vi "Check Can Uninit.vi"(8 "Error in":errorcluster, 10 "Actor in":refnum<class "Actor.lvclass">) -> (1 "Uninit":bool, 2 "Actor out":refnum<class "Actor.lvclass">)   [LabVIEW 2020, in "jettl.lvlib" / "Actor.lvlib"]
uses:
  Actor.lvlib
  Actor/Actor.lvclass
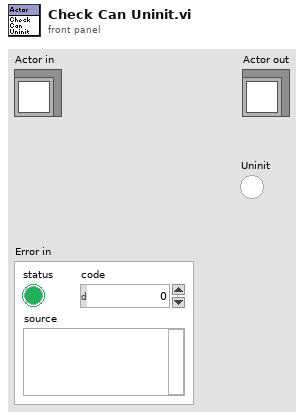
[diagram p1: front panel]
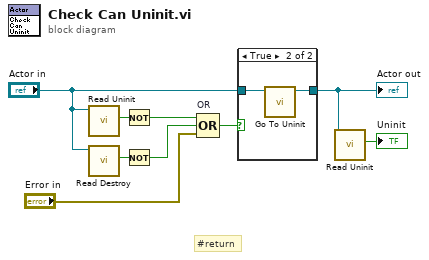
[diagram p0: block diagram]
diagram:
  # "#return"
  n1 = call-dynamic "Read Uninit.vi"("Actor in"="Actor in") -> ("Uninit"=w9:bool)  [unwired: 10 in]
  n2 = call-dynamic "Read Destroy.vi"("Actor in"="Actor in") -> ("Destroy"=w6:bool)  [unwired: 10 in]
  n3 = Not(x=w9) -> (.not. x?=w4:bool)
  n4 = Not(x=w6) -> (.not. x?=w3:bool)
  n5 = Compound Arithmetic op=OR "OR"(w4, w3, "Error in") -> (w8:bool)
  n6 = case shown="True" w8 {
    tunnel: "Actor in" -> [w10 w12]
    tunnel: [w10 w11] -> w1
    frame False {
    }
    frame True {
      n7 = call-dynamic "Go To Uninit.vi"("Actor in"=w12) -> ("Actor out"=w11:refnum<class "Actor.lvclass">)  [unwired: 10 in]
    }
  }
  "Actor out" <- w1
  n8 = call-dynamic "Read Uninit.vi"("Actor in"=w1) -> ("Uninit"=→"Uninit":bool)  [unwired: 10 in]
